vi "Rohde & Schwarz VNA Read Measurement.vi"(6 "Channel":i8=1 min=1 max=99 step=1, 7 "Rohde & Schwarz VNA":T1, 8 "error in (no error)":errorcluster, 11 "VISA Resource Name":refnum<visa-resource-name>) -> (0 "error out":errorcluster, 2 "Measurement (S11)":T2, 3 "dup VISA Resource Name":refnum<visa-resource-name>)   [LabVIEW 2011]
doc: "This VI for the HP 8753B is used to read the meausurement format.\n\n0 log magnitude\n1 phase\n2 delay\n3 Smith chart\n4 polar\n5 linear magnitude\n6 standing wave ratio\n7 real\n8 imaginary"
uses:
  TypeDefs/Rohde & Schwarz VNA Measurement.ctl
  TypeDefs/Rohde & Schwarz VNA Instrument Info.ctl
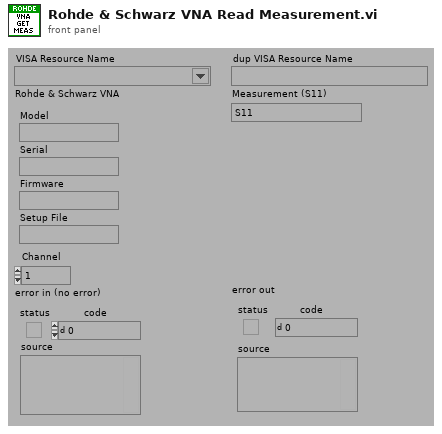
[diagram p1: front panel]
types:
  T1 = typedef "Rohde & Schwarz VNA Instrument Info.ctl" = cluster{"Model":string, "Serial":string, "Firmware":string, "Setup File":string}
  T2 = typedef "Rohde & Schwarz VNA Measurement.ctl" = enum32{"S11", "S12", "S21", "S22", "A1 Port 1 Source", "A1 Port 2 Source", "A2 Port 1 Source", "A2 Port 2 Source", "B1 Port 1 Source", "B1 Port 2 Source", "B2 Port 1 Source", "B2 Port 2 Source", "A1/A2 Port 1 Source", "A1/A2 Port 2 Source", "A1/B1 Port 1 Source", "A1/B1 Port 2 Source", "A1/B2 Port 1 Source", "A1/B2 Port 2 Source", "A2/A1 Port 1 Source", "A2/A1 Port 2 Source", "A2/B1 Port 1 Source", "A2/B1 Port 2 Source", "A2/B2 Port 1 Source", "A2/B2 Port 2 Source", "B1/A1 Port 1 Source", "B1/A1 Port 2 Source", "B1/A2 Port 1 Source", "B1/A2 Port 2 Source", "B1/B2 Port 1 Source", "B1/B2 Port 2 Source", "B2/A1 Port 1 Source", "B2/A1 Port 2 Source", "B2/A2 Port 1 Source", "B2/A2 Port 2 Source", "B2/B1 Port 1 Source", "B2/B1 Port 2 Source", "Z<-S11", "Z<-S12", "Z<-S21", "Z<-S22", "Y<-S11", "Y<-S12", "Y<-S21", "Y<-S22", "Z11", "Z12", "Z21", "Z22", "Y11", "Y12", "Y21", "Y22", "DC±1V", "DC±10V", "Unsupported"}
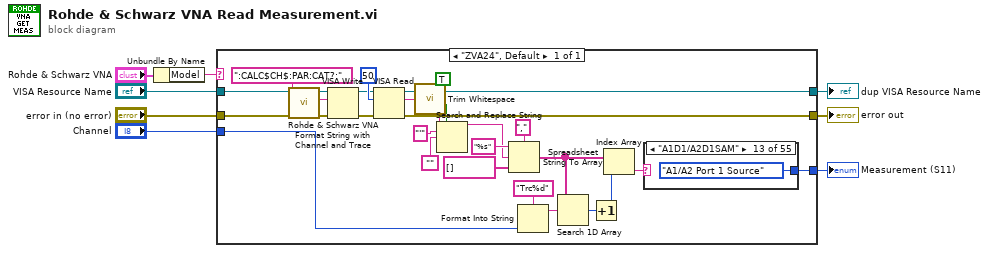
[diagram p0: block diagram]
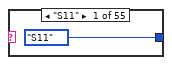
[diagram p2: hidden frame]
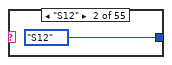
[diagram p3: hidden frame]
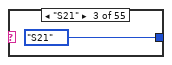
[diagram p4: hidden frame]
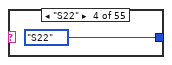
[diagram p5: hidden frame]
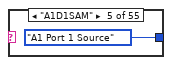
[diagram p6: hidden frame]
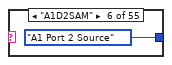
[diagram p7: hidden frame]
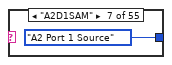
[diagram p8: hidden frame]
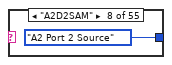
[diagram p9: hidden frame]
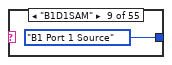
[diagram p10: hidden frame]
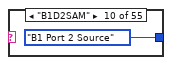
[diagram p11: hidden frame]
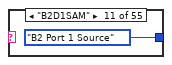
[diagram p12: hidden frame]
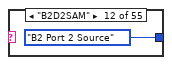
[diagram p13: hidden frame]
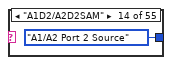
[diagram p14: hidden frame]
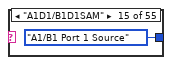
[diagram p15: hidden frame]
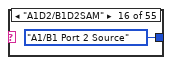
[diagram p16: hidden frame]
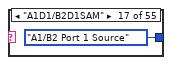
[diagram p17: hidden frame]
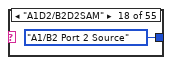
[diagram p18: hidden frame]
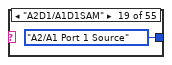
[diagram p19: hidden frame]
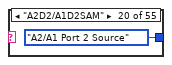
[diagram p20: hidden frame]
diagram:
  n1 = Unbundle By Name("Rohde & Schwarz VNA") -> ("Model"=w1:string)
  n2 = case shown="\"ZVA24\", Default" w1 {
    tunnel: "VISA Resource Name" -> [w28]
    tunnel: "error in (no error)" -> [w32]
    tunnel: [w30] -> w6
    tunnel: [w25] -> w5
    tunnel: [w29] -> w4
    tunnel: "Channel" -> [w20]
    frame "ZVA24", Default {
      n3 = call "Rohde & Schwarz VNA Format String with Channel and Trace.vi"("String"=":CALC$CH$:PAR:CAT?;") -> ("String Out"=w26:string)  [unwired: 2 in, 6 out]
      n4 = VISA Write(VISA resource name=w28, write buffer=w26, error in (no error)=w32) -> (VISA resource name out=w33:refnum<visa-resource-name>, error out=w31:errorcluster)  [unwired: 1 out]
      n5 = VISA Read(VISA resource name=w33, byte count=u32 50, error in (no error)=w31) -> (VISA resource name out=w29:refnum<visa-resource-name>, read buffer=w10:string, error out=w30:errorcluster)  [unwired: 1 out]
      n6 = call <vilib>:"Trim Whitespace.vi"("string"=w10) -> ("trimmed string"=w9:string)  [unwired: 1 in]
      n7 = Search and Replace String(replace all?=TRUE ("replace all? (F)"), input string=w9, search string="'", replace string="") -> (result string=w14:string)  [unwired: 1 in, 6 out]
      n8 = Spreadsheet String To Array(delimiter (Tab)=",", format string="%s" ("delimiter (Tab)"), spreadsheet string=w14, array type (2D Dbl)=string[] []) -> (array=w17:string[])
      n9 = Format Into String(format string="Trc%d", w20) -> (resulting string=w19:string)  [unwired: 2 in, 1 out]
      n10 = Search 1D Array(1D array=w17, element=w19) -> (index of element=w18:i32)  [unwired: 1 out]
      n11 = Increment(x=w18) -> (x+1=w16:i32)
      n12 = Index Array(array=w17, index=w16) -> (element=w15:string)
      n13 = case shown="\"A1D1/A2D1SAM\"" w15 {
        tunnel: [Rohde_&_Schwarz_VNA_Measurement."S11" ("Display Format") Rohde_&_Schwarz_VNA_Measurement."S12" ("Display Format") Rohde_&_Schwarz_VNA_Measurement."S21" ("Display Format") Rohde_&_Schwarz_VNA_Measurement."S22" ("Display Format") Rohde_&_Schwarz_VNA_Measurement."A1 Port 1 Source" ("Display Format") Rohde_&_Schwarz_VNA_Measurement."A1 Port 2 Source" ("Display Format") Rohde_&_Schwarz_VNA_Measurement."A2 Port 1 Source" ("Display Format") Rohde_&_Schwarz_VNA_Measurement."A2 Port 2 Source" ("Display Format") Rohde_&_Schwarz_VNA_Measurement."B1 Port 1 Source" ("Display Format") Rohde_&_Schwarz_VNA_Measurement."B1 Port 2 Source" ("Display Format") Rohde_&_Schwarz_VNA_Measurement."B2 Port 1 Source" ("Display Format") Rohde_&_Schwarz_VNA_Measurement."B2 Port 2 Source" ("Display Format") Rohde_&_Schwarz_VNA_Measurement."A1/A2 Port 1 Source" ("Display Format") Rohde_&_Schwarz_VNA_Measurement."A1/A2 Port 2 Source" ("Display Format") Rohde_&_Schwarz_VNA_Measurement."A1/B1 Port 1 Source" ("Display Format") Rohde_&_Schwarz_VNA_Measurement."A1/B1 Port 2 Source" ("Display Format") Rohde_&_Schwarz_VNA_Measurement."A1/B2 Port 1 Source" ("Display Format") Rohde_&_Schwarz_VNA_Measurement."A1/B2 Port 2 Source" ("Display Format") Rohde_&_Schwarz_VNA_Measurement."A2/A1 Port 1 Source" ("Display Format") Rohde_&_Schwarz_VNA_Measurement."A2/A1 Port 2 Source" ("Display Format") Rohde_&_Schwarz_VNA_Measurement."A2/B1 Port 1 Source" ("Display Format") Rohde_&_Schwarz_VNA_Measurement."A2/B1 Port 2 Source" ("Display Format") Rohde_&_Schwarz_VNA_Measurement."A2/B2 Port 1 Source" ("Display Format") Rohde_&_Schwarz_VNA_Measurement."A2/B2 Port 2 Source" ("Display Format") Rohde_&_Schwarz_VNA_Measurement."B1/A1 Port 1 Source" ("Display Format") Rohde_&_Schwarz_VNA_Measurement."B1/A1 Port 2 Source" ("Display Format") Rohde_&_Schwarz_VNA_Measurement."B1/A2 Port 1 Source" ("Display Format") Rohde_&_Schwarz_VNA_Measurement."B1/A2 Port 2 Source" ("Display Format") Rohde_&_Schwarz_VNA_Measurement."B1/B2 Port 1 Source" ("Display Format") Rohde_&_Schwarz_VNA_Measurement."B1/B2 Port 2 Source" ("Display Format") Rohde_&_Schwarz_VNA_Measurement."B2/A1 Port 1 Source" ("Display Format") Rohde_&_Schwarz_VNA_Measurement."B2/A1 Port 2 Source" ("Display Format") Rohde_&_Schwarz_VNA_Measurement."B2/A2 Port 1 Source" ("Display Format") Rohde_&_Schwarz_VNA_Measurement."B2/A2 Port 2 Source" ("Display Format") Rohde_&_Schwarz_VNA_Measurement."B2/B1 Port 1 Source" ("Display Format") Rohde_&_Schwarz_VNA_Measurement."B2/B1 Port 2 Source" ("Display Format") Rohde_&_Schwarz_VNA_Measurement."Z<-S11" ("Display Format") Rohde_&_Schwarz_VNA_Measurement."Z<-S12" ("Display Format") Rohde_&_Schwarz_VNA_Measurement."Z<-S21" ("Display Format") Rohde_&_Schwarz_VNA_Measurement."Z<-S22" ("Display Format") Rohde_&_Schwarz_VNA_Measurement."Y<-S11" ("Display Format") Rohde_&_Schwarz_VNA_Measurement."Y<-S12" ("Display Format") Rohde_&_Schwarz_VNA_Measurement."Y<-S21" ("Display Format") Rohde_&_Schwarz_VNA_Measurement."Y<-S22" ("Display Format") Rohde_&_Schwarz_VNA_Measurement."Z11" ("Display Format") Rohde_&_Schwarz_VNA_Measurement."Z12" ("Display Format") Rohde_&_Schwarz_VNA_Measurement."Z21" ("Display Format") Rohde_&_Schwarz_VNA_Measurement."Z22" ("Display Format") Rohde_&_Schwarz_VNA_Measurement."Y11" ("Display Format") Rohde_&_Schwarz_VNA_Measurement."Y12" ("Display Format") Rohde_&_Schwarz_VNA_Measurement."Y21" ("Display Format") Rohde_&_Schwarz_VNA_Measurement."Y22" ("Display Format") Rohde_&_Schwarz_VNA_Measurement."DC±1V" ("Display Format") Rohde_&_Schwarz_VNA_Measurement."DC±10V" ("Display Format") Rohde_&_Schwarz_VNA_Measurement."Unsupported" ("Display Format")] -> w25
        frame "S11" {
        }
        frame "S12" {
        }
        frame "S21" {
        }
        frame "S22" {
        }
        frame "A1D1SAM" {
        }
        frame "A1D2SAM" {
        }
        frame "A2D1SAM" {
        }
        frame "A2D2SAM" {
        }
        frame "B1D1SAM" {
        }
        frame "B1D2SAM" {
        }
        frame "B2D1SAM" {
        }
        frame "B2D2SAM" {
        }
        frame "A1D1/A2D1SAM" {
        }
        frame "A1D2/A2D2SAM" {
        }
        frame "A1D1/B1D1SAM" {
        }
        frame "A1D2/B1D2SAM" {
        }
        frame "A1D1/B2D1SAM" {
        }
        frame "A1D2/B2D2SAM" {
        }
        frame "A2D1/A1D1SAM" {
        }
        frame "A2D2/A1D2SAM" {
        }
        frame "A2D1/B1D1SAM" {
        }
        frame "A2D2/B1D2SAM" {
        }
        frame "A2D1/B2D1SAM" {
        }
        frame "A2D2/B2D2SAM" {
        }
        frame "B1D1/A1D1SAM" {
        }
        frame "B1D2/A1D2SAM" {
        }
        frame "B1D1/A2D1SAM" {
        }
        frame "B1D2/A2D2SAM" {
        }
        frame "B1D1/B2D1SAM" {
        }
        frame "B1D2/B2D2SAM" {
        }
        frame "B2D1/A1D1SAM" {
        }
        frame "B2D2/A1D2SAM" {
        }
        frame "B2D1/A2D1SAM" {
        }
        frame "B2D2/A2D2SAM" {
        }
        frame "B2D1/B1D1SAM" {
        }
        frame "B2D2/B1D2SAM" {
        }
        frame "Z-S11" {
        }
        frame "Z-S12" {
        }
        frame "Z-S21" {
        }
        frame "Z-S22" {
        }
        frame "Y-S11" {
        }
        frame "Y-S12" {
        }
        frame "Y-S21" {
        }
        frame "Y-S22" {
        }
        frame "Z11" {
        }
        frame "Z12" {
        }
        frame "Z21" {
        }
        frame "Z22" {
        }
        frame "Y11" {
        }
        frame "Y12" {
        }
        frame "Y21" {
        }
        frame "Y22" {
        }
        frame "DC±1V" {
        }
        frame "DC±10V" {
        }
        frame Default {
        }
      }
    }
  }
  "Measurement (S11)" <- w5
  "dup VISA Resource Name" <- w4
  "error out" <- w6
